vi "Reset VISA Device.vi"(8 "Error In":errorcluster, 11 "VISA resource name":refnum<visa-resource-name>) -> (0 "Error Out":errorcluster)   [LabVIEW 2014, in "LMH-LINX.lvlib" / "Device.lvlib"]
doc: "Reset LINX device by toggling DTR Lines"
uses:
  <vilib>/MakerHub/LINX/Private/Device/Device.lvlib
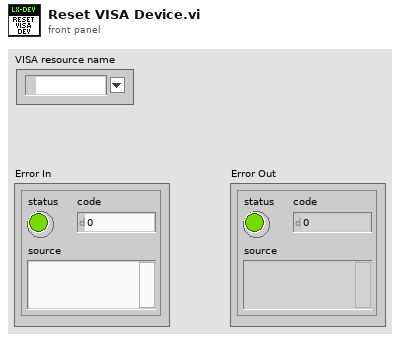
[diagram p1: front panel]
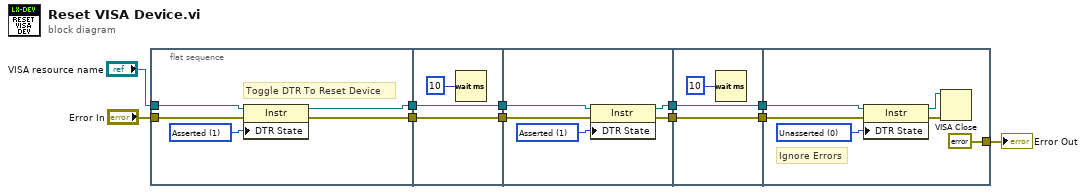
[diagram p0: block diagram]
diagram:
  n1 = flat-sequence {
    tunnel: "Error In" -> [w15]
    tunnel: "VISA resource name" -> [w14]
    tunnel: [w13] -> w4
    tunnel: [w12] -> w2
    tunnel: w4 -> [w19]
    tunnel: [w19] -> w3
    tunnel: w2 -> [w18]
    tunnel: [w18] -> w1
    tunnel: [w22] -> w11
    tunnel: [w21] -> w10
    tunnel: w3 -> [w23]
    tunnel: w1 -> [w20]
    tunnel: w11 -> [w26]
    tunnel: [w26] -> w9
    tunnel: w10 -> [w25]
    tunnel: [w25] -> w8
    tunnel: w9 -> [w30]
    tunnel: w8 -> [w29]
    tunnel: [errorcluster {"status"=FALSE, "code"=0, "source"=""} ("Error Out")] -> w5
    frame #0 {
      w16 = i16 1 items=["Unknown"=-1, "Unasserted"=0, "Asserted"=1] ("Serial Settings:Modem Line Settings:Line DTR State")
      # "Toggle DTR To Reset Device"
      n2 = property class="Instr"(reference=w14, error in=w15, "DTR State"=w16) -> (reference out=w13:refnum<visa-resource-name>, error out=w12:errorcluster)
    }
    frame #1 {
      n3 = Wait (ms)(milliseconds to wait=u32 10) -> ()  [unwired: 1 out]
    }
    frame #2 {
      w24 = i16 1 items=["Unknown"=-1, "Unasserted"=0, "Asserted"=1] ("Serial Settings:Modem Line Settings:Line DTR State")
      n4 = property class="Instr"(reference=w23, error in=w20, "DTR State"=w24) -> (reference out=w21:refnum<visa-resource-name>, error out=w22:errorcluster)
    }
    frame #3 {
      n5 = Wait (ms)(milliseconds to wait=u32 10) -> ()  [unwired: 1 out]
    }
    frame #4 {
      w31 = i16 0 items=["Unknown"=-1, "Unasserted"=0, "Asserted"=1] ("Serial Settings:Modem Line Settings:Line DTR State")
      # "Ignore Errors"
      n6 = property class="Instr"(reference=w29, error in=w30, "DTR State"=w31) -> (reference out=w32:refnum<visa-resource-name>, error out=w33:errorcluster)
      n7 = VISA Close(VISA resource name=w32, error in (no error)=w33) -> ()  [unwired: 1 out]
    }
  }
  "Error Out" <- w5
